vi "LinearScale.vi"(0 "RawInput":dbl, 5 "UnitsPlease Inputs":T1) -> (4 "UnitOutput":dbl)   [LabVIEW 2014]
panel:
  # "Andrew's Note: You should input a cluster of constants to this VI to make it more generic"
  # "Used to tell us which Potentiometer we are scaling"
  # "Inputs should be:\nin_min\nin_max\nout_min\nout_max\nand not specific to which they are"
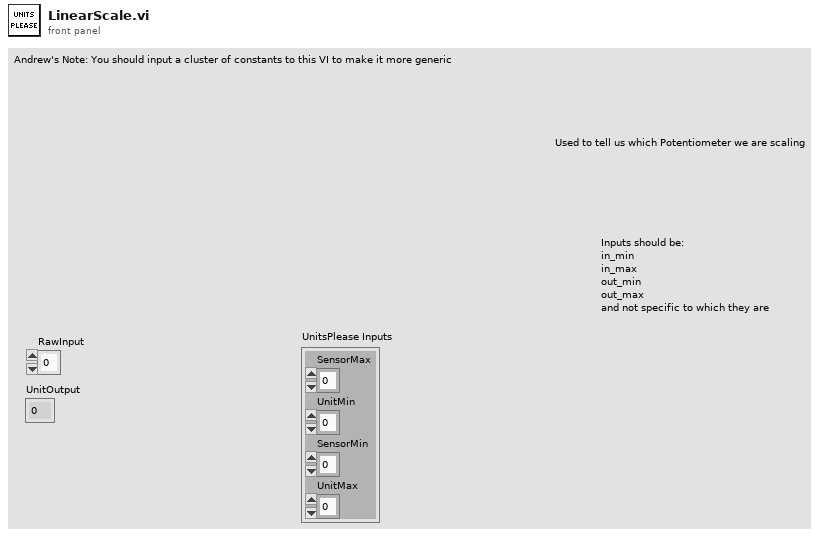
[diagram p1: front panel]
types:
  T1 = cluster{"SensorMax":dbl, "UnitMin":dbl, "SensorMin":dbl, "UnitMax":dbl}
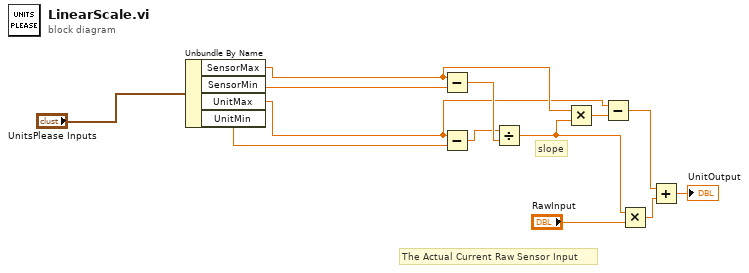
[diagram p0: block diagram]
diagram:
  # "slope"
  # "The Actual Current Raw Sensor Input"
  n1 = Unbundle By Name("UnitsPlease Inputs") -> ("SensorMax"=w5:dbl, "SensorMin"=w10:dbl, "UnitMax"=w2:dbl, "UnitMin"=w9:dbl)
  n2 = Subtract(x=w5, y=w10) -> (x-y=w8:dbl)
  n3 = Subtract(x=w2, y=w9) -> (x-y=w7:dbl)
  n4 = Divide(x=w7, y=w8) -> (x/y=w4:dbl)
  n5 = Multiply(x=w5, y=w4) -> (x*y=w3:dbl)
  n6 = Subtract(x=w2, y=w3) -> (x-y=w1:dbl)
  n7 = Multiply(x=w4, y="RawInput") -> (x*y=w13:dbl)
  n8 = Add(x=w1, y=w13) -> (x+y=→"UnitOutput":dbl)
